vi "PS35_GetSerNumber.vi"(0 "Control unit ID":i32=1 min=1 max=10, 1 "error in (no error)":errorcluster) -> (2 "Serial number":string, 3 "String length":i32, 4 "error out":errorcluster)   [LabVIEW 2020]
doc: "PS35_GetSerNumber.vi, created: 03.03.2009 alex; last change: 22.10.2019 alex;\n\n<B>FUNCTION:</B> \n\nRead serial number of the control unit.\n----------------------------------------------------------------------------------------\n<B>INPUT:</B>\n[I32] <B>Control unit ID:</B> control unit index. (Default=1, Range=1...10) \n[CLU] <B>error in</B>\n----------------------------------------------------------------------------------------\n<B>OUTPUT:</B>\n[CStr] <B>Serial number:</B> serial number of the control unit.\n[I32] <B>String length:</B> length of the string.\n[CLU] <B>error out</B>\n----------------------------------------------------------------------------------------\n<B>SUB-VIs:</B>\nPS35_GetReadError.vi\n----------------------------------------------------------------------------------------\n<B>EXT-Calls:</B>\nps35.dll (V2.01)\n----------------------------------------------------------------------------------------"
uses:
  ps35.dll
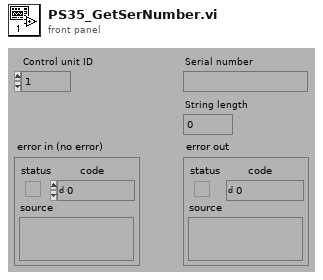
[diagram p1: front panel]
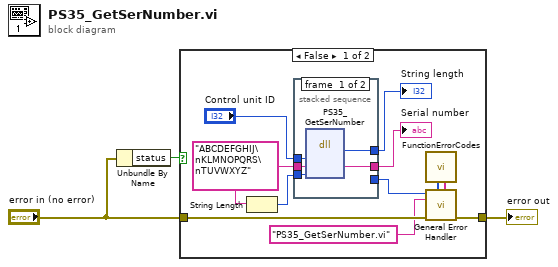
[diagram p0: block diagram]
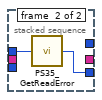
[diagram p2: hidden frame]
diagram:
  n1 = Unbundle By Name("error in (no error)") -> ("status"=w1:bool)
  n2 = case shown="False" w1 {
    tunnel: "error in (no error)" -> [w13 w22]
    tunnel: [w12 w22] -> w3
    frame False {
      w10 = "ABCDEFGHIJ\nKLMNOPQRS\nTUVWXYZ"
      n3 = String Length(string=w10) -> (length=w9:i32)
      n4 = stacked-sequence {
        tunnel: "Control unit ID" -> [w19 w21]
        tunnel: [w18 _] -> w11
        tunnel: w10 -> [w17 _]
        tunnel: w9 -> [w16 _]
        tunnel: [w15 _] -> w8
        tunnel: [_ w20] -> w7
        frame #0 {
          n5 = dll-call lib="C:/GEECS/Developers Version/source/Device Drivers/OwiSoft/OWISoftOEM/ps35/labview/lv82/ps35.dll" fn="PS35_GetSerNumber" label="PS35_Get\nSerNumber"("Index"=w19, "szString"=w17, "Length"=w16) -> ("Rückgabetyp"=w15:i32, "szString"=w18:string)  [unwired: 5 in, 2 out]
        }
        frame #1 {
          n6 = call "PS35_GetReadError.vi"("Control unit ID"=w21) -> ("Read error"=w20:i32)
        }
      }
      "Serial number" <- w11
      "String length" <- w8
      n7 = call "FunctionErrorCodes.vi"() -> ("[user-defined codes]"=w5:i32[], "[user-defined descriptions]"=w4:string[])  [unwired: 8 in]
      n8 = call <vilib>:"General Error Handler.vi"("[error code] (0)"=w7, "[user-defined codes]"=w5, "[user-defined descriptions]"=w4, "[error source] (\" \")"="PS35_GetSerNumber.vi" ("[error source] (\" \")"), "error in (no error)"=w13) -> ("error out"=w12:errorcluster)  [unwired: 6 in, 4 out]
    }
    frame True {
    }
  }
  "error out" <- w3
